vi "Test view.vi"(8 "error out":errorcluster, 11 "file (use dialog)":path) -> ()   [LabVIEW 2016]
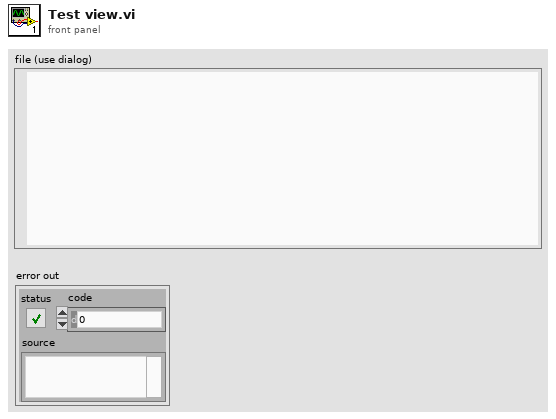
[diagram p1: front panel]
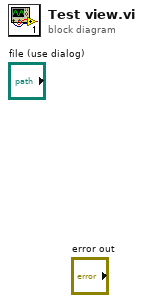
[diagram p0: block diagram]
diagram:
